vi "Write PmuImpairRptArray.vi"(8 "error in (no error)":errorcluster, 10 "PmuImpairRptArray":T1 {"Synx" format="%#_4g"}, 11 "OutputToFileBasePlugin in":refnum<class "OutputToFileBasePlugin.lvclass">) -> (0 "error out":errorcluster, 3 "OutputToFileBasePlugin out":refnum<class "OutputToFileBasePlugin.lvclass">)   [LabVIEW 2014, in "OutputToFilePlugins.lvlib" / "OutputToFileBasePlugin.lvclass"]
uses:
  OutputToFileBasePlugin.lvclass
  EventPlugins/EventPluginBaseClass/TypeDefs/clEvtReportArray.ctl
  EventPlugins/EventPluginBaseClass/TypeDefs/clEvtReport.ctl
  OutputToFileBasePlugin.lvclass/OutputToFileBasePlugin.ctl
  EventPlugins/EventPluginBaseClass/EventPluginBaseClass.lvclass
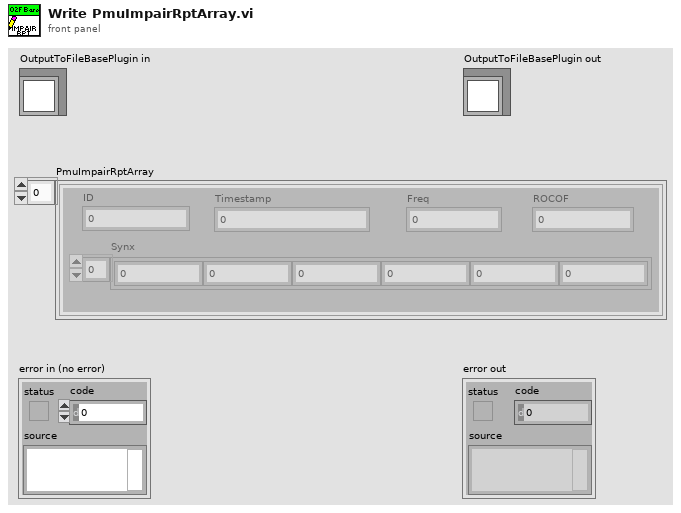
[diagram p1: front panel]
types:
  T1 = typedef "EventPlugins.lvlib/EventPluginBaseClass.lvclass/clEvtReportArray.ctl" = T2[]
  T2 = typedef "EventPlugins.lvlib/EventPluginBaseClass.lvclass/clEvtReport.ctl" = cluster{"Timestamp":dbl, "Synx":cdb[], "Freq":dbl, "ROCOF":dbl, "ID":i16}
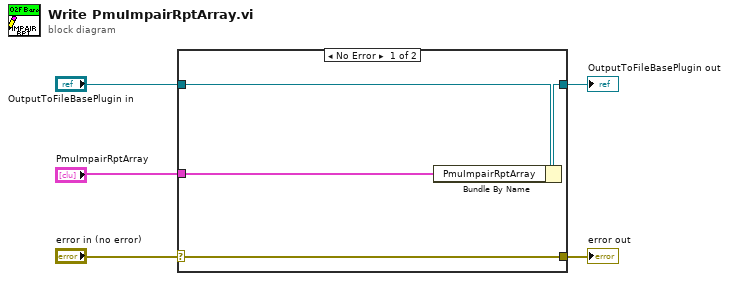
[diagram p0: block diagram]
diagram:
  n1 = case shown="No Error" "error in (no error)" {
    selector: "error in (no error)" -> [w9 w10]
    tunnel: [w9 w10] -> w4
    tunnel: [w8 w11] -> w2
    tunnel: "OutputToFileBasePlugin in" -> [w7 w11]
    tunnel: "PmuImpairRptArray" -> [w6 _]
    frame No Error {
      n2 = Bundle By Name(cluster=w7, "PmuImpairRptArray"=w6) -> (w8:refnum<class "OutputToFileBasePlugin.lvclass">)
    }
    frame Error {
    }
  }
  "error out" <- w4
  "OutputToFileBasePlugin out" <- w2
